vi "car_spec.vi"(11 "Car_name":string) -> ()   [LabVIEW 2015]
uses:
  rio_Global.vi
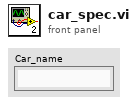
[diagram p1: front panel]
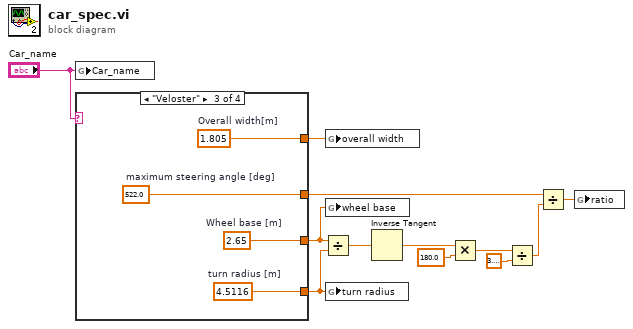
[diagram p0: block diagram]
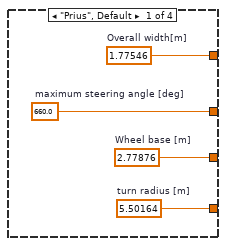
[diagram p2: hidden frame]
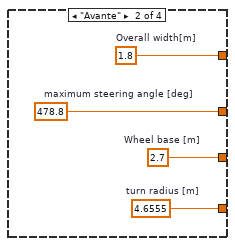
[diagram p3: hidden frame]
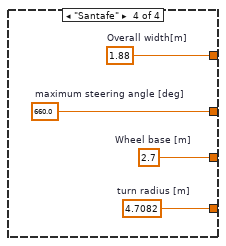
[diagram p4: hidden frame]
diagram:
  n1 = global write "rio_Global.vi" "Car_name"("Car_name") -> ()
  n2 = case shown="\"Veloster\"" "Car_name" {
    tunnel: [w16 w20 w24 w28] -> w7
    tunnel: [w15 w19 w23 w27] -> w8
    tunnel: [w14 w18 w22 w26] -> w9
    tunnel: [w13 w17 w21 w25] -> w11
    frame "Prius", Default {
      w14 = 1.77546  # Overall width[m]
      w16 = 660.0  # maximum steering angle [deg]
      w13 = 5.50164  # turn radius [m]
      w15 = 2.77876  # Wheel base [m]
    }
    frame "Avante" {
      w18 = 1.8  # Overall width[m]
      w20 = 478.8  # maximum steering angle [deg]
      w17 = 4.6555  # turn radius [m]
      w19 = 2.7  # Wheel base [m]
    }
    frame "Veloster" {
      w22 = 1.805  # Overall width[m]
      w24 = 522.0  # maximum steering angle [deg]
      w21 = 4.5116  # turn radius [m]
      w23 = 2.65  # Wheel base [m]
    }
    frame "Santafe" {
      w26 = 1.88  # Overall width[m]
      w28 = 660.0  # maximum steering angle [deg]
      w25 = 4.7082  # turn radius [m]
      w27 = 2.7  # Wheel base [m]
    }
  }
  n3 = Divide(x=w8, y=w11) -> (x/y=w1:dbl)
  n4 = global write "rio_Global.vi" "overall width"(w9) -> ()
  n5 = global write "rio_Global.vi" "wheel base"(w8) -> ()
  n6 = global write "rio_Global.vi" "turn radius"(w11) -> ()
  n7 = Inverse Tangent(1:w1) -> (0:w5:dbl)
  n8 = Multiply(x=w5, y=180.0) -> (x*y=w3:dbl)
  n9 = Divide(x=w3, y=3.141592653589793) -> (x/y=w6:dbl)
  n10 = Divide(x=w7, y=w6) -> (x/y=w10:dbl)
  n11 = global write "rio_Global.vi" "ratio"(w10) -> ()
